vi "InitDriver.vi"(8 "error in (no error)":errorcluster) -> (0 "error out":errorcluster)   [LabVIEW 2015, in "ESLSCDLL.lvlib"]
uses:
  ESLSCDLL.lvlib
  Globals.vi
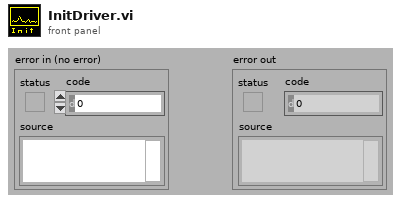
[diagram p1: front panel]
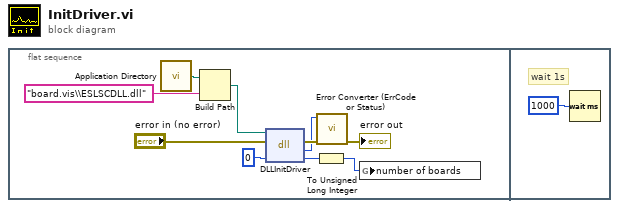
[diagram p0: block diagram]
diagram:
  n1 = flat-sequence {
    frame #0 {
      n2 = call <vilib>:"Application Directory.vi"() -> ("Application Directory"=w3:path)
      n3 = Build Path(base path=w3, name or relative path="board.vis\\ESLSCDLL.dll") -> (appended path=w1:path)
      n4 = dll-call lib="C:/ENTW/PCIE/LV64/board.vis/ESLSCDLL.dll" fn="DLLInitDriver" ("lwlscdll.dll:DLLCCDDrvInit")(path in=w1, error in="error in (no error)", "number_of_boards"=u8 0) -> (error out=w8:errorcluster, "es_status_codes"=w7:i32, "number_of_boards"=w5:u8)  [unwired: 1 in, 1 out]
      n5 = To Unsigned Long Integer(number=w5) -> (unsigned 32bit integer=w4:u32)
      n6 = call "Error Converter (ErrCode or Status).vi"("error in (no error)"=w8, "error code"=w7) -> ("error out"=→"error out":errorcluster)  [unwired: 9 in]
      n7 = global write "Globals.vi" "number of boards"(w4) -> ()
    }
    frame #1 {
      # "wait 1s"
      n8 = Wait (ms)(milliseconds to wait=u32 1000) -> ()  [unwired: 1 out]
    }
  }
